vi "CreateError.vi"(6 "AdditionalText":string, 7 "Data":variant, 8 "ErrorIn":errorcluster caption="Error In", 9 "Text":string, 10 "ErrorCode":i32) -> (0 "ErrorOut":errorcluster caption="Error Out")   [LabVIEW 2018, in "ErrorCreationExecution.lvclass"]
uses:
  <userlib>/_express/CustomErrorCreator/ErrorCreationExecution/ErrorCreationExecution.lvclass
  <userlib>/_express/CustomErrorCreator/ErrorCreationTypes/ErrorCreationMGI/ErrorCreationMGI.lvclass
  C:/Program Files (x86)/National Instruments/LabVIEW 2018/user.lib/_express/CustomErrorCreator/ErrorCreationExecution/ErrorCreationExecution.lvclass
  <userlib>/_express/CustomErrorCreator/ErrorCreationExecution/ErrorCreationType.vi
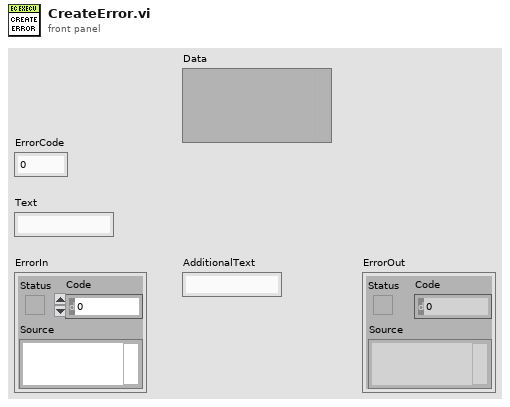
[diagram p1: front panel]
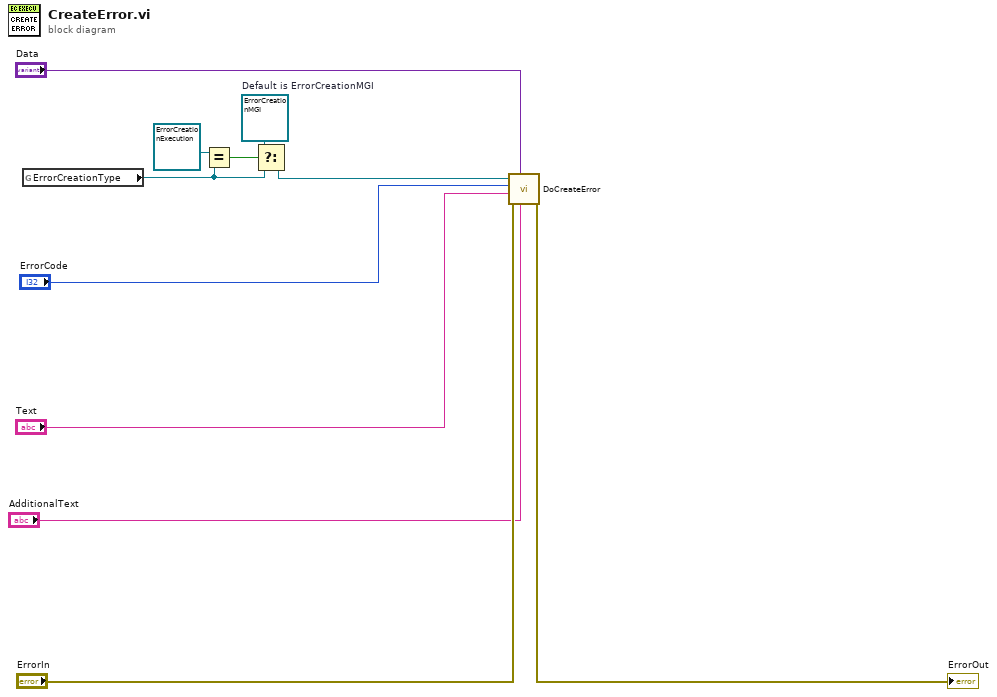
[diagram p0: block diagram]
diagram:
  w1 = refnum<class "ErrorCreationMGI.lvclass"> refnum  # Default is ErrorCreationMGI
  n1 = global read "ErrorCreationType.vi" "ErrorCreationType"() -> (w3:refnum<class "ErrorCreationExecution.lvclass">)
  n2 = Equal?(x=refnum<class "ErrorCreationExecution.lvclass"> refnum ("ErrorCreationExecution"), y=w3) -> (x = y?=w4:bool)
  n3 = Select(t=w1, s=w4, f=w3) -> (s? t:f=w2:refnum<class "ErrorCreationExecution.lvclass">)
  n4 = call-dynamic "DoCreateError.vi"("AdditionalText"="AdditionalText", "Data"="Data", "ErrorIn"="ErrorIn", "Text"="Text", "ErrorCode"="ErrorCode", "ObjectIn"=w2) -> ("ErrorOut"=→"ErrorOut":errorcluster)  [unwired: 4 in, 1 out]
